vi "Polling Core.vi"(8 "Error In":errorcluster, 11 "BNT_ULx-MCSV in":refnum<class "BNT_ULx-MCSV.lvclass">) -> (0 "Error Out":errorcluster, 3 "BNT_ULx-MCSV out":refnum<class "BNT_ULx-MCSV.lvclass">)   [LabVIEW 2020, in "BNT_ULx.lvlib" / "BNT_ULx-MCSV.lvclass"]
uses:
  BNT_ULx-MCSV.lvclass
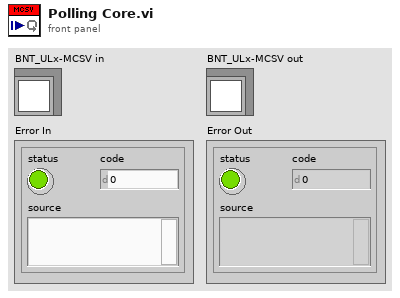
[diagram p1: front panel]
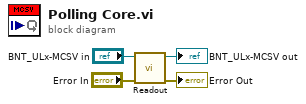
[diagram p0: block diagram]
diagram:
  n1 = call "Readout.vi"("Error In"="Error In", "BNT_ULx-MCSV in"="BNT_ULx-MCSV in") -> ("Error Out"=→"Error Out":errorcluster, "BNT_ULx-MCSV out"=→"BNT_ULx-MCSV out":refnum<class "BNT_ULx-MCSV.lvclass">)  [unwired: 7 in, 1 out]
